vi "Build Header String.vi"(9 "Section":string, 10 "Strings[]":string[](array[string]), 11 "Header in":string) -> (3 "Header out":string)   [LabVIEW 2015]
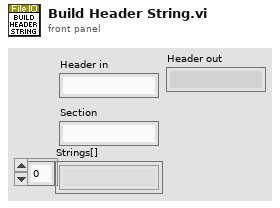
[diagram p1: front panel]
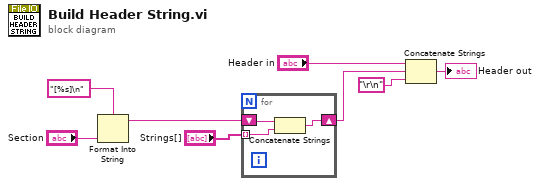
[diagram p0: block diagram]
diagram:
  n1 = Format Into String(format string="[%s]\n", "Section") -> (resulting string=w3:string)  [unwired: 2 in, 1 out]
  n2 = for {
    shift-right: [w11] -> w6
    shift-left: w3 -> [w10]
    tunnel: "Strings[]" -> [w9] mode=indexing
    n3 = Concatenate Strings(w10, w9) -> (w11:string)
  }
  n4 = Concatenate Strings("Header in", w6, "\r\n") -> (→"Header out":string)
